vi "Validate From Module Connection Information.vi"(8 "error in":errorcluster, 10 "module connection information in":T1[](array[typedef]), 11 "routing and faulting in":T3 format="%.0x") -> (0 "error out":errorcluster, 2 "module connection information out":T1[](array[typedef]), 3 "routing and faulting out":T3 format="%.0x")   [LabVIEW 2020, in "Routing and Faulting Scripting.lvlib"]
uses:
  Routing and Faulting Scripting.lvlib
  Types/Module Information.ctl
  Shared/Routing and Faulting Hardware API/Types/Possible Connections for Endpoint.ctl
  <vilib>/NI VeriStand/Custom Device API/Custom Device Item Ref.ctl
  Shared/Routing and Faulting Hardware API/Routing and Faulting Hardware API.lvlib
  <vilib>/NI VeriStand/Custom Device API/Custom Device API.lvlib
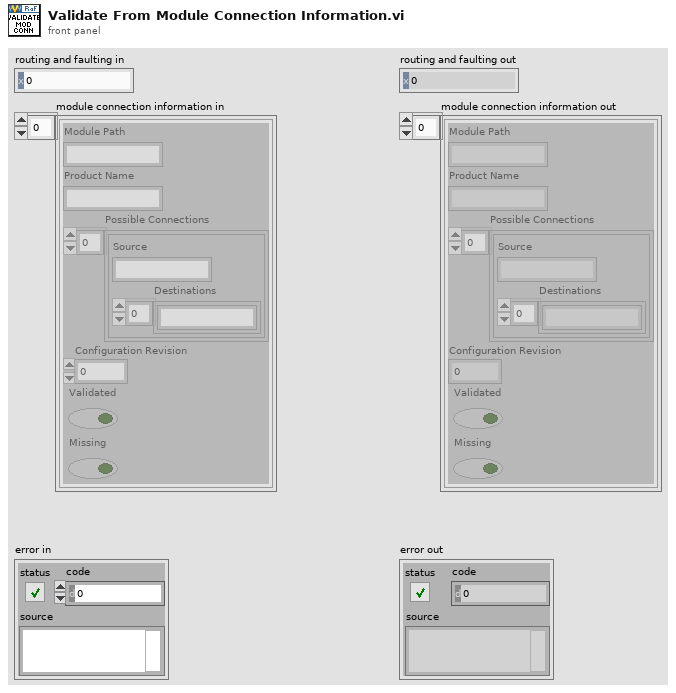
[diagram p1: front panel]
types:
  T1 = typedef "Routing and Faulting Scripting.lvlib/Module Information.ctl" = cluster{"Module Path":string, "Product Name":string, "Possible Connections":T2[], "Configuration Revision":u32, "Validated":bool, "Missing":bool}
  T2 = typedef "Routing and Faulting Hardware API.lvlib/Possible Connections for Endpoint.ctl" = cluster{"Source":string, "Destinations":string[]}
  T3 = typedef "Custom Device API.lvlib/Custom Device Item Ref.ctl" = u64
  T4 = typedef "Routing and Faulting Scripting.lvlib/Validation Information.ctl" = cluster{"Missing Modules":variant, "Module Connection Map":variant, "Unused Modules":variant}
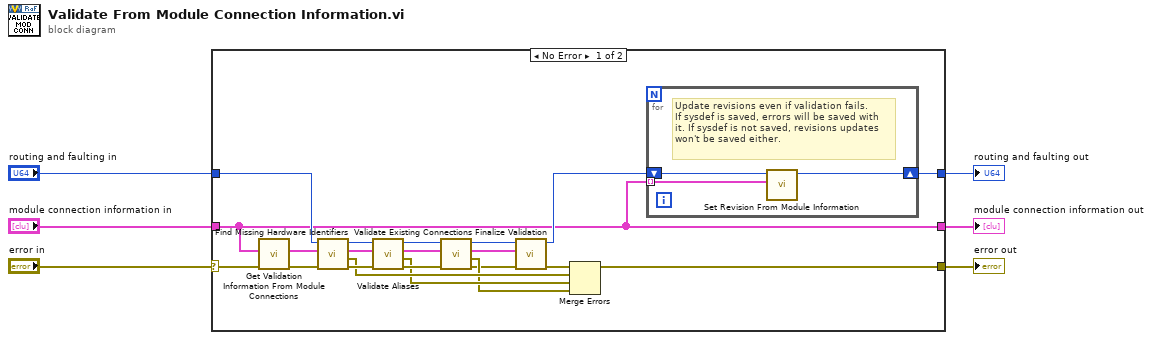
[diagram p0: block diagram]
diagram:
  n1 = case shown="No Error" "error in" {
    selector: "error in" -> [w19 w33]
    tunnel: "module connection information in" -> [w7 w31]
    tunnel: [w10 w33] -> w5
    tunnel: "routing and faulting in" -> [w21 w32]
    tunnel: [w8 w32] -> w2
    tunnel: [w7 w31] -> w1
    frame No Error {
      n2 = call "Get Validation Information From Module Connections.vi"("error in"=w19, "module connection information"=w7) -> ("error out"=w20:errorcluster, "validation information"=w18:T4)  [unwired: 8 in]
      n3 = call "Find Missing Hardware Identifiers.vi"("error in"=w20, "validation information in"=w18, "routing and faulting in"=w21) -> ("error out"=w27:errorcluster, "identifier errors"=w17:errorcluster[], "validation information out"=w23:T4, "routing and faulting out"=w26:T3)  [unwired: 5 in]
      n4 = call "Validate Aliases.vi"("error in"=w27, "validation information in"=w23, "routing and faulting in"=w26) -> ("error out"=w25:errorcluster, "aliases errors"=w16:errorcluster[], "validation information out"=w22:T4, "routing and faulting out"=w24:T3)  [unwired: 5 in]
      n5 = call "Validate Existing Connections.vi"("error in"=w25, "validation information in"=w22, "routing and faulting in"=w24) -> ("error out"=w14:errorcluster, "connection errors"=w15:errorcluster[], "validation information out"=w11:T4, "routing and faulting out"=w12:T3)  [unwired: 5 in]
      n6 = call "Finalize Validation.vi"("error in"=w14, "validation information"=w11, "routing and faulting in"=w12) -> ("error out"=w13:errorcluster, "routing and faulting out"=w9:T3)  [unwired: 7 in]
      n7 = Merge Errors(w13, w17, w16, w15) -> (w10:errorcluster)
      n8 = for {
        shift-right: [w29] -> w8
        shift-left: w9 -> [w30]
        tunnel: w7 -> [w28] mode=indexing
        # "Update revisions even if validation fails.\nIf sysdef is saved, errors will be saved with\nit. If sysdef is not saved, revisions updates\nwon't be saved either."
        n9 = call "Set Revision From Module Information.vi"("module information"=w28, "routing and faulting in"=w30) -> ("routing and faulting out"=w29:T3)  [unwired: 8 in, 1 out]
      }
    }
    frame Error {
    }
  }
  "error out" <- w5
  "routing and faulting out" <- w2
  "module connection information out" <- w1
